vi "validate even number.vi"(11 "Number":i32) -> (3 "Even":bool)   [LabVIEW 2014]
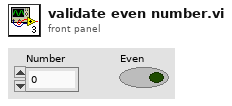
[diagram p1: front panel]
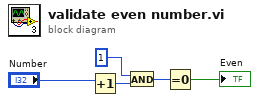
[diagram p0: block diagram]
diagram:
  n1 = Increment(x="Number") -> (x+1=w5:i32)
  n2 = And(x=1, y=w5) -> (x .and. y?=w3:i32)
  n3 = Equal To 0?(x=w3) -> (x = 0?=→"Even":bool)
